vi "send rel move to focus stage.vi"(8 "error in (no error)":errorcluster, 11 "Autofocus in":refnum<class "Autofocus.lvclass">) -> (0 "error out":errorcluster, 3 "Autofocus out":refnum<class "Autofocus.lvclass">)   [LabVIEW 2012, in "Autofocus.lvclass"]
uses:
  Autofocus.lvclass
  <vilib>/Distrio/Murmex/GenericMessage/GenericMessage.lvclass
  Autofocus.lvclass/Autofocus.ctl
  <vilib>/Distrio/Murmex/Message/Message.lvclass
  <vilib>/Distrio/Murmex/Murmex/Murmex.lvclass
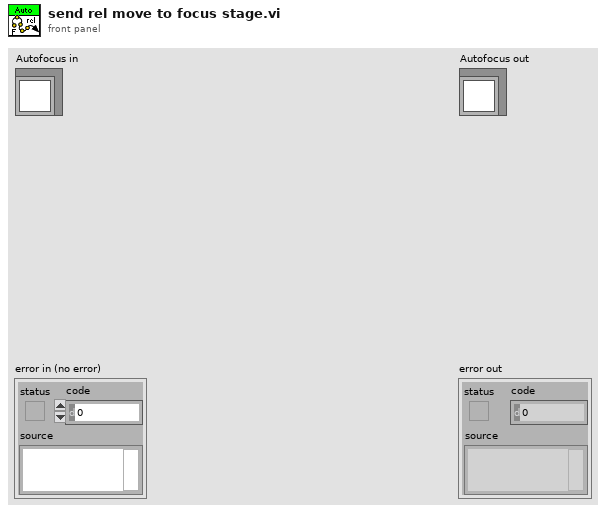
[diagram p1: front panel]
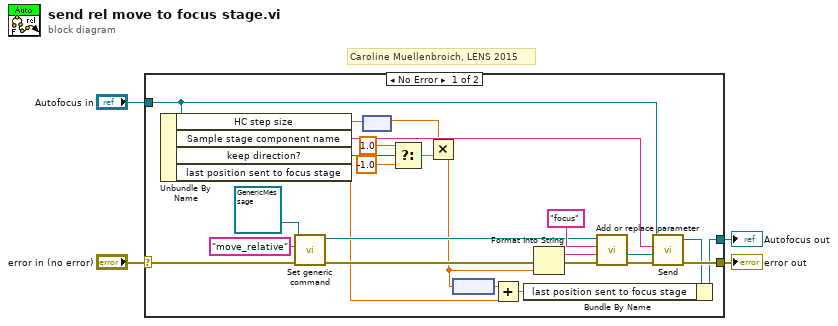
[diagram p0: block diagram]
diagram:
  # "Caroline Muellenbroich, LENS 2015"
  n1 = case shown="No Error" "error in (no error)" {
    selector: "error in (no error)" -> [w20 w31]
    tunnel: [w23 w31] -> w3
    tunnel: [w14 w30] -> w1
    tunnel: "Autofocus in" -> [w18 w30]
    frame No Error {
      n2 = Unbundle By Name(w18) -> ("HC step size"=w29:dbl[unit], "Sample stage component name"=w17:string, "keep direction?"=w13:bool, "last position sent to focus stage"=w5:dbl[unit])
      n3 = call <vilib>:"Set generic command.vi"("error in (no error)"=w20, "generic command"="move_relative" ("command string"), "GenericMessage in"=refnum<class "GenericMessage.lvclass"> refnum ("Murmex.lvlib:GenericMessage")) -> ("error out"=w19:errorcluster, "GenericMessage out"=w16:refnum<class "GenericMessage.lvclass">)  [unwired: 7 in]
      n4 = node(w29) -> (w10:dbl)
      n5 = Select(t=1.0, s=w13, f=-1.0) -> (s? t:f=w9:dbl)
      n6 = Multiply(x=w10, y=w9) -> (x*y=w7:dbl)
      n7 = node(w7) -> (w6:dbl[unit])
      n8 = Add(x=w6, y=w5) -> (x+y=w8:dbl[unit])
      n9 = Format Into String(error in=w19, w7) -> (resulting string=w25:string, error out=w24:errorcluster)  [unwired: 2 in]
      n10 = call <vilib>:"Add or replace parameter.vi"("error in (no error)"=w24, "value"=w25, "name"="focus", "Message in"=w16) -> ("error out"=w27:errorcluster, "Message out"=w28:refnum<class "GenericMessage.lvclass">)  [unwired: 6 in]
      n11 = call <vilib>:"Send.vi"("error in (no error)"=w27, "Message"=w28, "recipient"=w17, "Murmex in"=w18) -> ("error out"=w23:errorcluster, "Murmex out"=w15:refnum<class "Autofocus.lvclass">)  [unwired: 6 in]
      n12 = Bundle By Name(cluster=w15, "last position sent to focus stage"=w8) -> (w14:refnum<class "Autofocus.lvclass">)
    }
    frame Error {
    }
  }
  "error out" <- w3
  "Autofocus out" <- w1
